vi "InitCSMs(backup).vi"(8 "error in":errorcluster) -> (0 "error out":errorcluster, 2 "CSMs":string[](array[string]))   [LabVIEW 2017]
uses:
  Chain1.vi
  Chain2.vi
  Chain3.vi
  CSM-Testcase.lvlib
  src/user.lib/_NEVSTOP/Communicable State Machine(CSM)/Communicable State Machine.lvlib
panel:
  out "Waited (ms)":u32
  out "CSMs Left":string[](array[string])
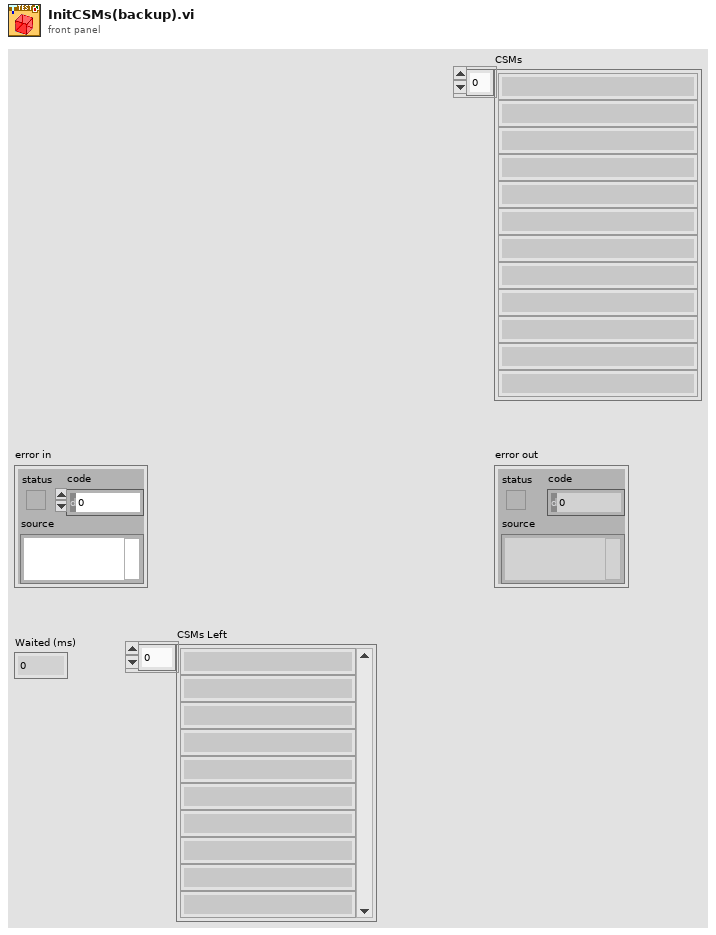
[diagram p1: front panel]
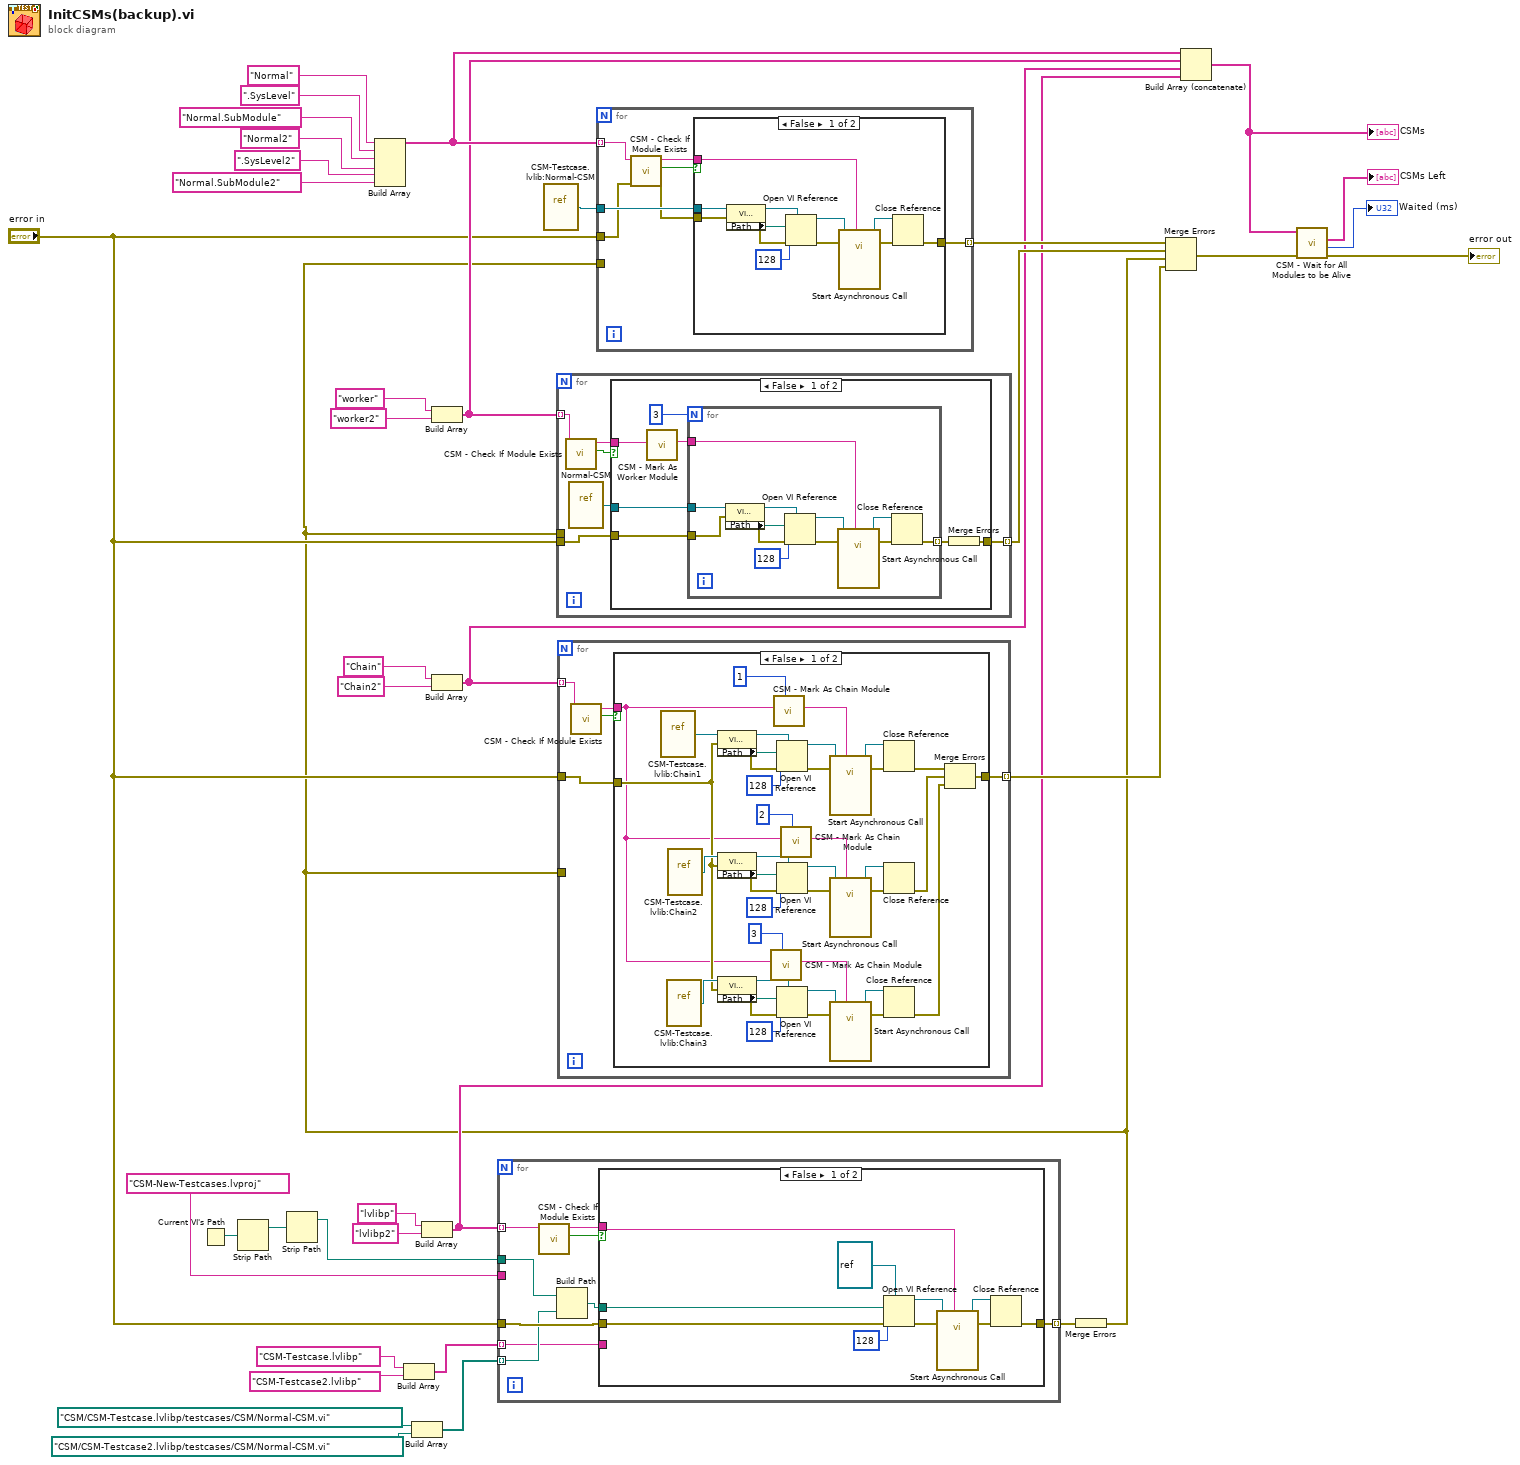
[diagram p0: block diagram]
diagram:
  n1 = Current VI's Path() -> (path=w34:path)
  n2 = Strip Path(path=w34) -> (stripped path=w35:path)  [unwired: 1 out]
  n3 = Strip Path(path=w35) -> (stripped path=w36:path)  [unwired: 1 out]
  n4 = Build Array("Normal" ("Name (\"\" to Use UUID)"), ".SysLevel" ("Name (\"\" to Use UUID)"), "Normal.SubModule" ("Name (\"\" to Use UUID)"), "Normal2" ("Name (\"\" to Use UUID)"), ".SysLevel2" ("Name (\"\" to Use UUID)"), "Normal.SubModule2" ("Name (\"\" to Use UUID)")) -> (w30:string[])
  n5 = Build Array("CSM-Testcase.lvlibp" ("Name of build specification (if empty: build all)"), "CSM-Testcase2.lvlibp" ("Name of build specification (if empty: build all)")) -> (w8:string[])
  n6 = Build Array(path "CSM/CSM-Testcase.lvlibp/testcases/CSM/Normal-CSM.vi" ("vi path"), path "CSM/CSM-Testcase2.lvlibp/testcases/CSM/Normal-CSM.vi" ("vi path")) -> (w11:path[])
  n7 = Build Array("lvlibp" ("Name (\"\" to Use UUID)"), "lvlibp2" ("Name (\"\" to Use UUID)")) -> (w14:string[])
  n8 = Build Array("worker" ("Name (\"\" to Use UUID)"), "worker2" ("Name (\"\" to Use UUID)")) -> (w20:string[])
  n9 = Build Array("Chain" ("Name (\"\" to Use UUID)"), "Chain2" ("Name (\"\" to Use UUID)")) -> (w17:string[])
  n10 = for {
    tunnel: "CSM-New-Testcases.lvproj" ("name or relative path") -> [_]
    tunnel: w36 -> [w41]
    tunnel: w14 -> [w43] mode=indexing
    tunnel: w11 -> [w42] mode=indexing
    tunnel: w8 -> [w39] mode=indexing
    tunnel: "error in" -> [w46]
    tunnel: [w45] -> w33 mode=indexing
    n11 = call "CSM - Check If Module Exists.vi"("CSM Name"=w43) -> ("Exist?"=w47:bool, "CSM Name (Dup)"=w44:string)  [unwired: 8 in, 1 out]
    n12 = Build Path(base path=w41, name or relative path=w42) -> (appended path=w40:path)
    n13 = case shown="False" w47 {
      tunnel: [w57 w58] -> w45
      tunnel: w40 -> [w48 _]
      tunnel: w44 -> [w50 _]
      tunnel: w46 -> [w49 w58]
      tunnel: w39 -> [_ _]
      frame False {
        n14 = Open VI Reference(type specifier VI Refnum (for type only)=refnum<vi> refnum ("reference out"), vi path=w48, options=128, error in (no error)=w49) -> (vi reference=w53:refnum<vi>, error out=w55:errorcluster)  [unwired: 2 in]
        n15 = call-by-ref "Start Asynchronous Call"(reference=w53, error in=w55, "Name (\"\" to Use UUID)"=w50) -> (reference out=w52:refnum<vi>, error out=w54:errorcluster)  [unwired: 11 in]
        n16 = Close Reference(reference=w52, error in (no error)=w54) -> (error out=w57:errorcluster)
      }
      frame True {
      }
    }
  }
  n17 = vi-ref "CSM-Testcase.lvlib:Normal-CSM.vi"() -> (w26:refnum<vi>)
  n18 = Merge Errors(w33) -> (w1:errorcluster)
  n19 = for {
    tunnel: w20 -> [w60] mode=indexing
    tunnel: "error in" -> [w64]
    tunnel: [w61] -> w32 mode=indexing
    tunnel: w1 -> [_]
    n20 = call "CSM - Check If Module Exists.vi"("CSM Name"=w60) -> ("Exist?"=w63:bool, "CSM Name (Dup)"=w62:string)  [unwired: 8 in, 1 out]
    n21 = vi-ref "Normal-CSM.vi"() -> (w59:refnum<vi>)
    n22 = case shown="False" w63 {
      tunnel: w59 -> [w71 _]
      tunnel: [w65 w84] -> w61
      tunnel: w64 -> [w67 w84]
      tunnel: w62 -> [w66 _]
      frame False {
        n23 = call "CSM - Mark As Worker Module.vi"("CSM Name"=w66) -> ("CSM Name (Marked As Worker)"=w68:string)  [unwired: 9 in]
        n24 = for {
          N: 3 -> [_]
          tunnel: w71 -> [w75]
          tunnel: w68 -> [w74]
          tunnel: [w73] -> w69 mode=indexing
          tunnel: w67 -> [w72]
          n25 = property class="VI (strict)"(reference=w75, error in=w72) -> (reference out=w81:refnum<vi>, error out=w79:errorcluster, "Path"=w78:path)
          n26 = Open VI Reference(type specifier VI Refnum (for type only)=w81, vi path=w78, options=128, error in (no error)=w79) -> (vi reference=w77:refnum<vi>, error out=w82:errorcluster)  [unwired: 2 in]
          n27 = call-by-ref "Start Asynchronous Call"(reference=w77, error in=w82, "Name (\"\" to Use UUID)"=w74) -> (reference out=w76:refnum<vi>, error out=w80:errorcluster)  [unwired: 11 in]
          n28 = Close Reference(reference=w76, error in (no error)=w80) -> (error out=w73:errorcluster)
        }
        n29 = Merge Errors(w69) -> (w65:errorcluster)
      }
      frame True {
      }
    }
  }
  n30 = for {
    tunnel: w17 -> [w85] mode=indexing
    tunnel: "error in" -> [w89]
    tunnel: [w87] -> w38 mode=indexing
    tunnel: w1 -> [_]
    n31 = call "CSM - Check If Module Exists.vi"("CSM Name"=w85) -> ("Exist?"=w88:bool, "CSM Name (Dup)"=w86:string)  [unwired: 8 in, 1 out]
    n32 = case shown="False" w88 {
      tunnel: [w92 w129] -> w87
      tunnel: w89 -> [w91 w129]
      tunnel: w86 -> [w90 _]
      frame False {
        n33 = vi-ref "CSM-Testcase.lvlib:Chain1.vi"() -> (w128:refnum<vi>)
        n34 = vi-ref "CSM-Testcase.lvlib:Chain3.vi"() -> (w110:refnum<vi>)
        n35 = vi-ref "CSM-Testcase.lvlib:Chain2.vi"() -> (w111:refnum<vi>)
        n36 = property class="VI (strict)"(reference=w128, error in=w91) -> (reference out=w125:refnum<vi>, error out=w123:errorcluster, "Path"=w122:path)
        n37 = property class="VI (strict)"(reference=w111, error in=w91) -> (reference out=w114:refnum<vi>, error out=w116:errorcluster, "Path"=w117:path)
        n38 = property class="VI (strict)"(reference=w110, error in=w91) -> (reference out=w107:refnum<vi>, error out=w105:errorcluster, "Path"=w104:path)
        n39 = call "CSM - Mark As Chain Module.vi"("Order"=3, "CSM Name"=w90) -> ("CSM Name (Marked As Chain)"=w98:string)  [unwired: 8 in]
        n40 = call "CSM - Mark As Chain Module.vi"("Order"=1, "CSM Name"=w90) -> ("CSM Name (Marked As Chain)"=w96:string)  [unwired: 8 in]
        n41 = Open VI Reference(type specifier VI Refnum (for type only)=w125, vi path=w122, options=128, error in (no error)=w123) -> (vi reference=w121:refnum<vi>, error out=w126:errorcluster)  [unwired: 2 in]
        n42 = Open VI Reference(type specifier VI Refnum (for type only)=w114, vi path=w117, options=128, error in (no error)=w116) -> (vi reference=w118:refnum<vi>, error out=w113:errorcluster)  [unwired: 2 in]
        n43 = Open VI Reference(type specifier VI Refnum (for type only)=w107, vi path=w104, options=128, error in (no error)=w105) -> (vi reference=w103:refnum<vi>, error out=w108:errorcluster)  [unwired: 2 in]
        n44 = call "CSM - Mark As Chain Module.vi"("Order"=2, "CSM Name"=w90) -> ("CSM Name (Marked As Chain)"=w97:string)  [unwired: 8 in]
        n45 = call-by-ref "Start Asynchronous Call"(reference=w121, error in=w126, "Name (\"\" to Use UUID)"=w96) -> (reference out=w120:refnum<vi>, error out=w124:errorcluster)  [unwired: 11 in]
        n46 = call-by-ref "Start Asynchronous Call"(reference=w118, error in=w113, "Name (\"\" to Use UUID)"=w97) -> (reference out=w119:refnum<vi>, error out=w115:errorcluster)  [unwired: 11 in]
        n47 = call-by-ref "Start Asynchronous Call"(reference=w103, error in=w108, "Name (\"\" to Use UUID)"=w98) -> (reference out=w102:refnum<vi>, error out=w106:errorcluster)  [unwired: 11 in]
        n48 = Close Reference(reference=w120, error in (no error)=w124) -> (error out=w101:errorcluster)
        n49 = Close Reference(reference=w119, error in (no error)=w115) -> (error out=w100:errorcluster)
        n50 = Close Reference(reference=w102, error in (no error)=w106) -> (error out=w99:errorcluster)
        n51 = Merge Errors(w101, w100, w99) -> (w92:errorcluster)
      }
      frame True {
      }
    }
  }
  n52 = for {
    tunnel: w26 -> [w136]
    tunnel: w30 -> [w132] mode=indexing
    tunnel: [w135] -> w31 mode=indexing
    tunnel: "error in" -> [w134]
    tunnel: w1 -> [_]
    n53 = call "CSM - Check If Module Exists.vi"("Error In"=w134, "CSM Name"=w132) -> ("error out"=w133:errorcluster, "Exist?"=w130:bool, "CSM Name (Dup)"=w131:string)  [unwired: 7 in]
    n54 = case shown="False" w130 {
      tunnel: w136 -> [w140 _]
      tunnel: [w139 w149] -> w135
      tunnel: w133 -> [w138 w149]
      tunnel: w131 -> [w137 _]
      frame False {
        n55 = property class="VI (strict)"(reference=w140, error in=w138) -> (reference out=w146:refnum<vi>, error out=w144:errorcluster, "Path"=w143:path)
        n56 = Open VI Reference(type specifier VI Refnum (for type only)=w146, vi path=w143, options=128, error in (no error)=w144) -> (vi reference=w142:refnum<vi>, error out=w147:errorcluster)  [unwired: 2 in]
        n57 = call-by-ref "Start Asynchronous Call"(reference=w142, error in=w147, "Name (\"\" to Use UUID)"=w137) -> (reference out=w141:refnum<vi>, error out=w145:errorcluster)  [unwired: 11 in]
        n58 = Close Reference(reference=w141, error in (no error)=w145) -> (error out=w139:errorcluster)
      }
      frame True {
      }
    }
  }
  n59 = Merge Errors(w31, w32, w1, w38) -> (w7:errorcluster)
  n60 = Build Array (concatenate)(w30, w20, w17, w14) -> (w6:string[])
  "CSMs" <- w6
  n61 = call "CSM - Wait for All Modules to be Alive.vi"("Error In"=w7, "CSM Names"=w6) -> ("error out"=→"error out":errorcluster, "Waited (ms)"=→"Waited (ms)":u32, "CSMs Left"=→"CSMs Left":string[])  [unwired: 7 in]
